vi "Release.vi"(8 "error in (no error)":errorcluster, 11 "YP03-60_Z in":refnum<class "YP03-60_Z.lvclass">) -> (0 "error out":errorcluster)   [LabVIEW 2020, in "PowerControl.lvlib" / "YP03-60_Z.lvclass"]
uses:
  YP03-60_Z.lvclass
  VirtualPower/VirtualPower.lvclass
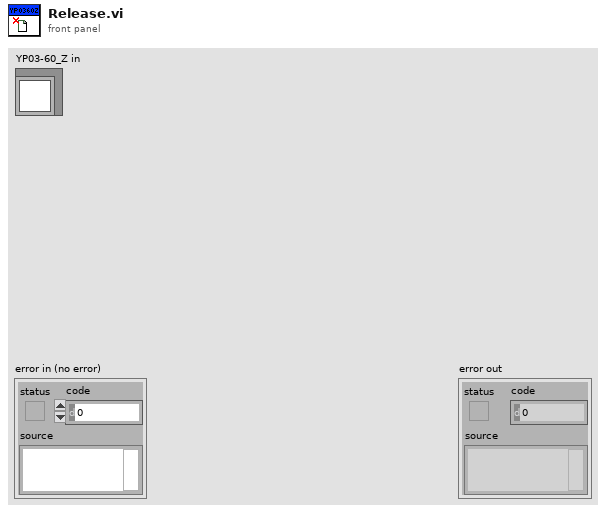
[diagram p1: front panel]
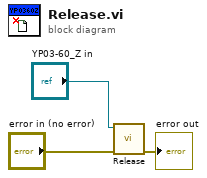
[diagram p0: block diagram]
diagram:
  n1 = call-parent "Release.vi"("error in (no error)"="error in (no error)", "VirtualPower in"="YP03-60_Z in") -> ("error out"=→"error out":errorcluster)  [unwired: 9 in]
